vi "读取connectID.vi"(8 "error in (no error)":errorcluster caption="错误输入（无错误）", 11 "data_inter输入":refnum<class "data_inter.lvclass">) -> (0 "error out":errorcluster caption="错误输出", 2 "connectID":refnum<k5>, 3 "data_inter输出":refnum<class "data_inter.lvclass">)   [LabVIEW 2016, in "潮位站数据传输.lvlib" / "data_inter.lvclass"]
uses:
  data_inter.lvclass
  data_inter.lvclass/data_inter.ctl
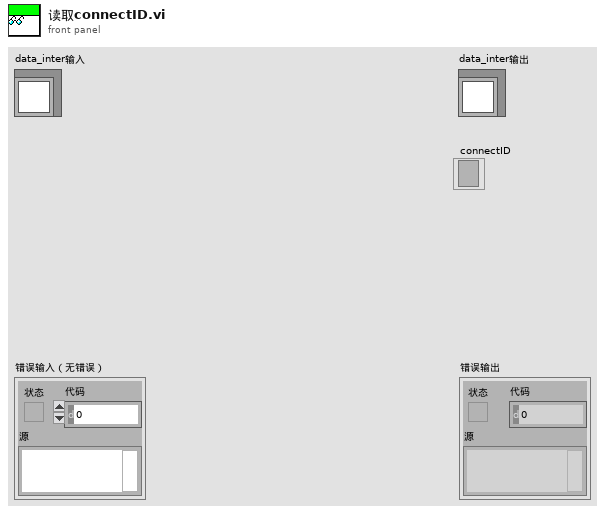
[diagram p1: front panel]
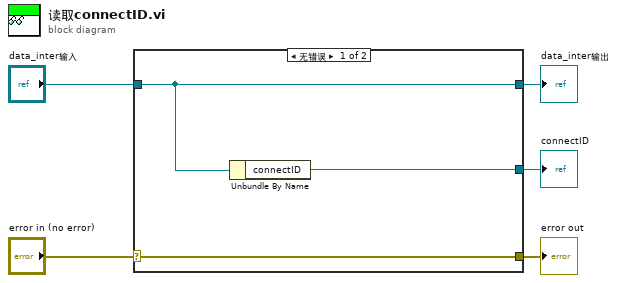
[diagram p0: block diagram]
diagram:
  n1 = case shown="无错误" "error in (no error)" {
    selector: "error in (no error)" -> [w8 w9]
    tunnel: [w8 w9] -> w4
    tunnel: [w7 w10] -> w2
    tunnel: "data_inter输入" -> [w7 w10]
    tunnel: [w6 _] -> w1
    frame No Error {
      n2 = Unbundle By Name(w7) -> ("connectID"=w6:refnum<k5>)
    }
    frame Error {
    }
  }
  "error out" <- w4
  "data_inter输出" <- w2
  "connectID" <- w1
